vi "12 - Design Pattern - Flaky Delegator Design Pattern with dotNET.vi"() -> ()   [LabVIEW 2012]
uses:
  System.Windows.Forms
panel:
  in  ".NET Button":refnum<k24>(container)
  out "Increment to 5 to exit":i32
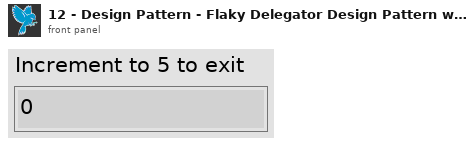
[diagram p1: front panel]
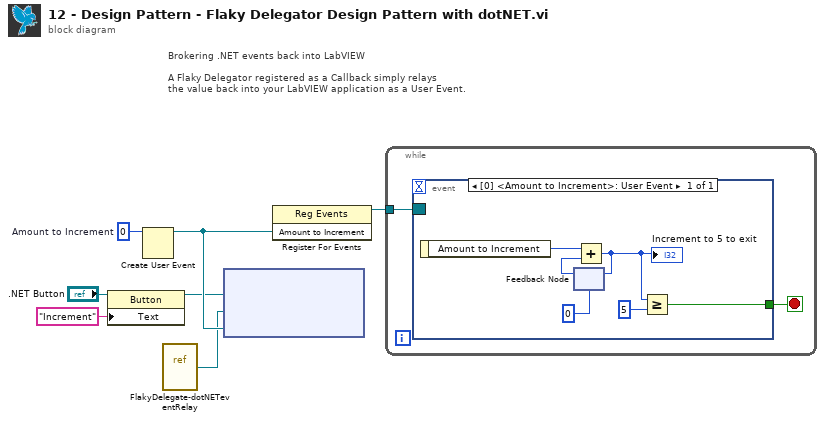
[diagram p0: block diagram]
diagram:
  w7 = 0  # Amount to Increment
  # "Brokering .NET events back into LabVIEW\n\nA Flaky Delegator registered as a Callback simply relays\nthe value back into your LabVIEW application as a User Event."
  n1 = property class="Button"(reference=".NET Button", "Text"="Increment") -> (reference out=w1:refnum<k24>)  [unwired: 1 in, 1 out]
  n2 = Create User Event(user event datatype=w7) -> (user event=w6:refnum<user-event>)  [unwired: 1 in, 1 out]
  n3 = vi-ref "FlakyDelegate-dotNETeventRelay.vi"() -> ("vi reference"=w4:refnum<vi>)
  n4 = node(w1, w4, w6) -> ()  [unwired: 2 in, 2 out]
  n5 = register-events(w6) -> (reference out=w5:refnum<event-registration>)  [unwired: 2 in, 1 out]
  n6 = while {
    tunnel: w5 -> [w8]
    stop <- w9 stop-if-true
    n7 = event shown="[0] <Amount to Increment>: User Event" {
      selector: w8 -> [_]
      dyn-events: _ -> [_]
      timeout: _ -> [_]
      tunnel: [w14] -> w9
      event User Event {
        n8 = event-data() -> ("Amount to Increment"=w12:i32)  [unwired: 1 in]
        n9 = feedback #1(0) -> (w13:i32)
        n10 = Add(x=w12, y=w13) -> (x+y=w11:i32)
        "Increment to 5 to exit" <- w11
        n11 = feedback-in #1(w11) -> ()
        n12 = Greater Or Equal?(x=w11, y=5) -> (x >= y?=w14:bool)
      }
    }
  }
